vi "JAUS Transport Layer.vi"() -> ()   [LabVIEW 2009]
uses:
  cRIO/Functional Global Variables/Actions for FG's.ctl
  Support Files/JUDP Write Queue Element.ctl
  Support Files/JUDP Read Queue Element.ctl
  Support Files/Address.ctl
  Support Files/LogData.ctl
panel:
  out "UDP Write Loop":bool
  out "UDP Read Loop":bool
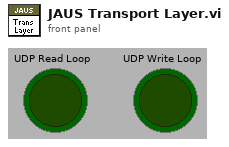
[diagram p1: front panel]
types:
  T1 = typedef "Actions for FG's.ctl" = enum16{"Read", "Write"}
  T2 = typedef "JUDP Write Queue Element.ctl" = cluster{"Encoded JAUS Message":string, "Destination ID":u32}
  T3 = typedef "JUDP Read Queue Element.ctl" = cluster{"Payload":string, "Sender ID":T4, "Command Code":u16}
  T4 = typedef "Address.ctl" = cluster{"Subsystem Id":u16, "Node Id":u8, "Component Id":u8}
  T5 = cluster{"QueryType":u8, "Type":u16, "COP Identification":string}
  T6 = typedef "LogData.ctl" = cluster{"Time Stamp":timestamp, "JAUS Message":string, "Command Code":string}
  T7 = typedef "UDP Base.ctl" = cluster{"UDP Session":refnum<k16>, "UDP Socket Params":T8}
  T8 = typedef "UDP Socket Params.ctl" = cluster{"Local Port":u16, "Read Timeout":i32, "Write Timeout":i32}
  T9 = typedef "UDP Network Location.ctl" = cluster{"IP Address":string, "Port":u16}
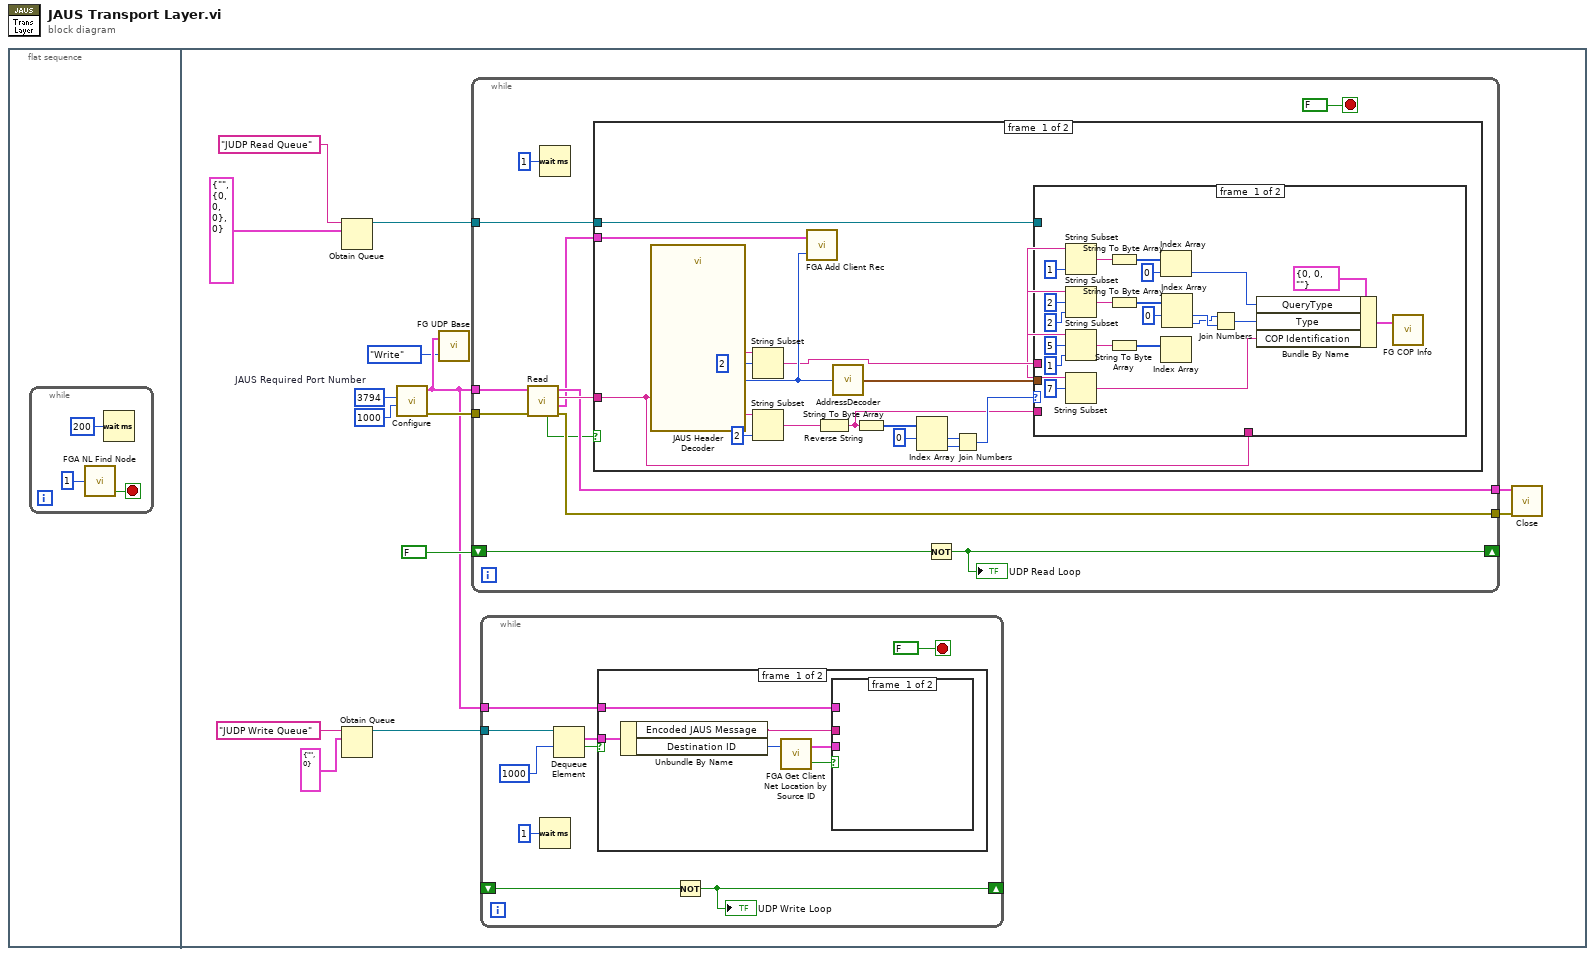
[diagram p0: block diagram]
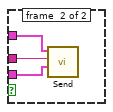
[diagram p2: hidden frame]
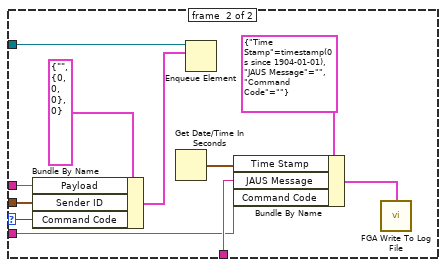
[diagram p4: hidden frame]
diagram:
  n1 = flat-sequence {
    frame #0 {
      n2 = while {
        stop <- w2 stop-if-true
        n3 = call "FGA NL Find Node.vi"("Node ID"=u8 1) -> ("Record Exists?"=w2:bool)  [unwired: 2 in, 2 out]
        n4 = Wait (ms)(milliseconds to wait=u32 200) -> ()  [unwired: 1 out]
      }
    }
    frame #1 {
      w13 = u16 3794  # JAUS Required Port Number
      n5 = Obtain Queue(name (unnamed)="JUDP Read Queue", element data type=T3 {"Payload"="", "Sender ID"={"Subsystem Id"=0, "Node Id"=0, "Component Id"=0}, "Command Code"=0} ("Receive FSM Queue Element")) -> (queue out=w15:refnum<queue>)  [unwired: 3 in, 2 out]
      n6 = Obtain Queue(name (unnamed)="JUDP Write Queue", element data type=T2 {"Encoded JAUS Message"="", "Destination ID"=0} ("Cluster")) -> (queue out=w8:refnum<queue>)  [unwired: 3 in, 2 out]
      n7 = call "Configure.vi"("Read Timeout"=1000, "Local Port"=w13) -> ("error out"=w14:errorcluster, "UDP Base out"=w5:T7)  [unwired: 8 in]
      n8 = call "FG UDP Base.vi"("FG Action (Read)"=Actions_for_FG's."Write", "UDP Base in"=w5) -> ()  [unwired: 1 out]
      n9 = while {
        tunnel: w15 -> [w47]
        tunnel: w5 -> [w45]
        tunnel: w14 -> [w46]
        tunnel: [w43] -> w11
        tunnel: [w42] -> w10
        shift-right: [w40] -> _
        shift-left: FALSE ("stop") -> [w41]
        stop <- FALSE stop-if-true
        n10 = call "Read.vi"("error in (no error)"=w46, "UDP Base in"=w45) -> ("error out"=w42:errorcluster, "Network Location"=w38:T9, "Receive Data"=w44:string, "UDP Base out"=w43:T7, "Timeout"=w39:bool)  [unwired: 4 in, 1 out]
        n11 = Wait (ms)(milliseconds to wait=u32 1) -> ()  [unwired: 1 out]
        n12 = case shown="False" w39 {
          tunnel: w47 -> [w54 _]
          tunnel: w44 -> [w49 _]
          tunnel: w38 -> [w55 _]
          frame #0 {
            n13 = call "JAUS Header Decoder.vi"("Encoded JAUS Message"=w49) -> ("Source ID (80-95)"=w53:u32, "Payload"=w57:string)  [unwired: 13 in, 12 out]
            n14 = String Subset(string=w57, offset (0)=2) -> (substring=w51:string)  [unwired: 1 in]
            n15 = String Subset(string=w57, length (rest)=2 ("length (rest)")) -> (substring=w58:string)  [unwired: 1 in]
            n16 = call "FGA Add Client Rec.vi"("ID"=w53, "Network Location"=w55) -> ()  [unwired: 1 in, 1 out]
            n17 = Reverse String(1:w58) -> (0:w48:string)
            n18 = call "AddressDecoder.vi"("Address"=w53) -> ("Address Cluster"=w52:T4)
            n19 = String To Byte Array(string=w48) -> (unsigned byte array=w63:u8[])
            n20 = Index Array(array=w63, index #1=0 ("index")) -> (element #1=w61:u8, element #2=w60:u8)  [unwired: 1 in]
            n21 = Join Numbers(hi=w61, lo=w60) -> ((hi.lo)=w50:u16)
            n22 = case shown="4B00" w50 {
              selector: w50 -> [_ w88]
              tunnel: w54 -> [_ w96]
              tunnel: w52 -> [_ w95]
              tunnel: w51 -> [w75 w94]
              tunnel: w49 -> [_ w89]
              tunnel: w48 -> [_ w87]
              frame #0 {
                n23 = String Subset(string=w75, length (rest)=1 ("length (rest)")) -> (substring=w85:string)  [unwired: 1 in]
                n24 = String Subset(string=w75, offset (0)=2, length (rest)=2 ("length (rest)")) -> (substring=w84:string)
                n25 = String Subset(string=w75, offset (0)=5, length (rest)=1 ("length (rest)")) -> (substring=w76:string)
                n26 = String Subset(string=w75, offset (0)=7) -> (substring=w72:string)  [unwired: 1 in]
                n27 = String To Byte Array(string=w85) -> (unsigned byte array=w71:u8[])
                n28 = String To Byte Array(string=w84) -> (unsigned byte array=w67:u8[])
                n29 = String To Byte Array(string=w76) -> (unsigned byte array=w79:u8[])
                n30 = Index Array(array=w71, index=0) -> (element=w69:u8)
                n31 = Index Array(array=w79) -> ()  [unwired: 1 in, 1 out]
                n32 = Index Array(array=w67, index #1=0 ("index")) -> (element #1=w66:u8, element #2=w65:u8)  [unwired: 1 in]
                n33 = Join Numbers(hi=w65, lo=w66) -> ((hi.lo)=w64:u16)
                n34 = Bundle By Name(cluster=T5 {"QueryType"=0, "Type"=0, "COP Identification"=""} ("COP Info in"), "QueryType"=w69, "Type"=w64, "COP Identification"=w72) -> (w73:T5)
                n35 = call "FG COP Info.vi"("COP Info in"=w73) -> ()  [unwired: 1 in, 1 out]
              }
              frame #1 {
                n36 = Bundle By Name(cluster=T3 {"Payload"="", "Sender ID"={"Subsystem Id"=0, "Node Id"=0, "Component Id"=0}, "Command Code"=0} ("element"), "Payload"=w94, "Sender ID"=w95, "Command Code"=w88) -> (w92:T3)
                n37 = Get Date/Time In Seconds() -> (seconds since 1Jan1904=w90:timestamp)
                n38 = Enqueue Element(queue=w96, element=w92) -> ()  [unwired: 2 in, 3 out]
                n39 = Bundle By Name(cluster=T6 {"Time Stamp"=timestamp(0 s since 1904-01-01), "JAUS Message"="", "Command Code"=""} ("LogData"), "Time Stamp"=w90, "JAUS Message"=w89, "Command Code"=w87) -> (w86:T6)
                n40 = call "FGA Write To Log File.vi"("LogData"=w86) -> ()
              }
            }
          }
          frame #1 {
          }
        }
        n41 = Not(x=w41) -> (.not. x?=w40:bool)
        "UDP Read Loop" <- w40
      }
      n42 = while {
        shift-right: [w25] -> _
        shift-left: _ -> [w26]
        tunnel: w8 -> [w24]
        tunnel: w5 -> [w21]
        stop <- FALSE stop-if-true
        n43 = Wait (ms)(milliseconds to wait=u32 1) -> ()  [unwired: 1 out]
        n44 = Dequeue Element(queue=w24, timeout in ms (-1)=1000) -> (element=w22:T2, timed out?=w23:bool)  [unwired: 1 in, 2 out]
        n45 = case shown="False" w23 {
          tunnel: w22 -> [w31 _]
          tunnel: w21 -> [w32 _]
          frame #0 {
            n46 = Unbundle By Name(w31) -> ("Encoded JAUS Message"=w30:string, "Destination ID"=w29:u32)
            n47 = call "FGA Get Client Net Location by Source ID.vi"("ID"=w29) -> ("Record Exists?"=w28:bool, "Network Location"=w27:T9)  [unwired: 1 in]
            n48 = case shown="True" w28 {
              tunnel: w32 -> [_ w35]
              tunnel: w30 -> [_ w34]
              tunnel: w27 -> [_ w33]
              frame #0 {
              }
              frame #1 {
                n49 = call "Send.vi"("Destination Location"=w33, "Send Data"=w34, "UDP Base in"=w35) -> ()  [unwired: 6 in, 3 out]
              }
            }
          }
          frame #1 {
          }
        }
        n50 = Not(x=w26) -> (.not. x?=w25:bool)
        "UDP Write Loop" <- w25
      }
      n51 = call "Close.vi"("error in (no error)"=w10, "Cluster of class private data"=w11) -> ()  [unwired: 9 in, 1 out]
    }
  }
